vi "Encoder Motor.vi"() -> ()   [LabVIEW 2020]
uses:
  <vilib>/DAQmx/read.llb/DAQmx Read (Counter DBL 1Chan 1Samp).vi
  <vilib>/DAQmx/write.llb/DAQmx Write (Counter Frequency 1Chan 1Samp).vi
  <vilib>/DAQmx/create/channels.llb/DAQmx Create Channel (CI-Position-Angular Encoder).vi
  <vilib>/DAQmx/create/channels.llb/DAQmx Create Channel (CO-Pulse Generation-Frequency).vi
  <vilib>/DAQmx/configure/timing.llb/DAQmx Timing (Implicit).vi
  <vilib>/DAQmx/miscellaneous.llb/DAQmx Fill In Error Info.vi
  <resource>/objmgr/daqmx.rc
panel:
  out "Duty Cycle":dbl
  out "Gearbox RPM":dbl
  out "Within Range":bool
  out "Waveform Chart":dbl(graph)=3538.0740745250973
  in  "Encoder Input Counter":tag="Dev1/ctr1"
  in  "PWM Output counter":tag="Dev1/ctr0"
  out "Motor RPM":dbl
  in  "Desired RPM":dbl
  in  "stop":bool
  in  "PWM output terminal":tag="/Dev1/PFI0"
  in  "Encoder B input":tag="/Dev1/PFI9"
  in  "Encoder A input":tag="/Dev1/PFI8"
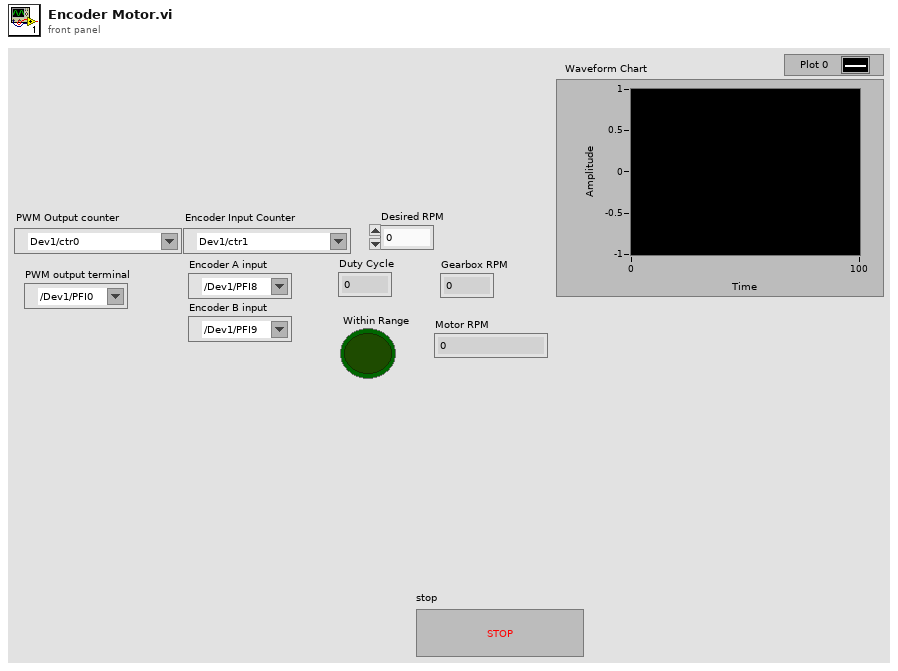
[diagram p1: front panel]
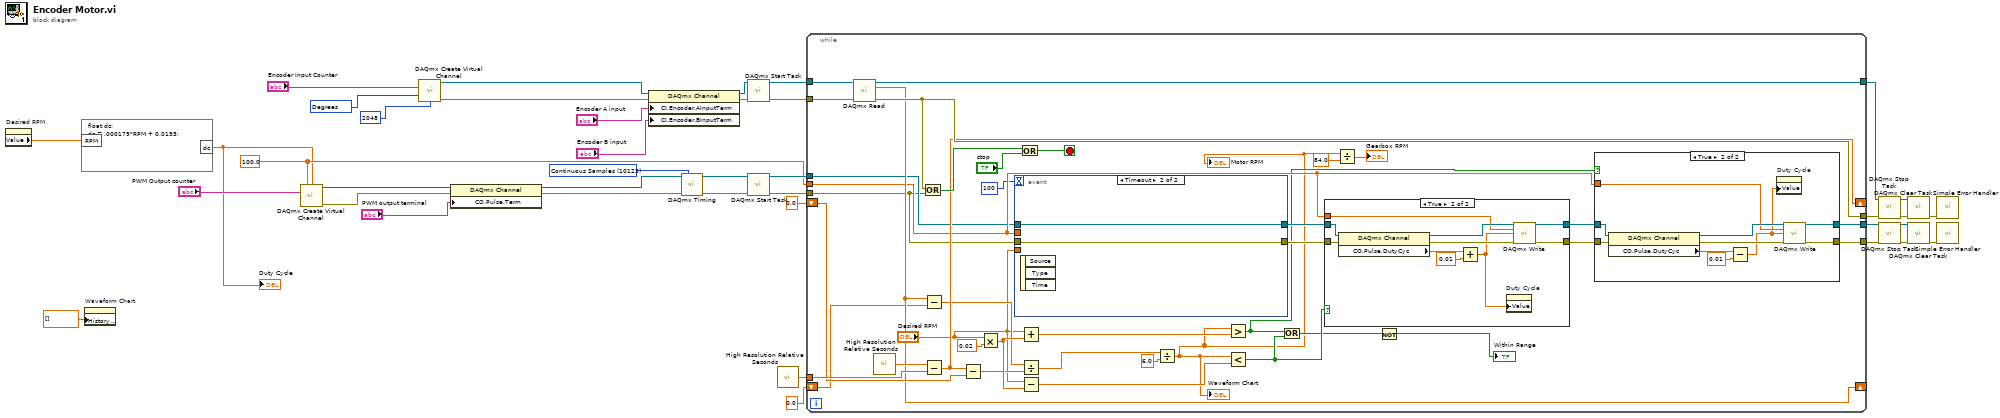
[diagram p0: block diagram]
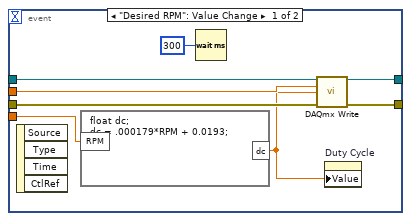
[diagram p4: hidden frame]
diagram:
  w8 = 10146 items=["Degrees"=10146, "Radians"=10273, "Ticks"=10304, "From Custom Scale"=10065] ("units")
  w14 = 10123 items=["Finite Samples"=10178, "Continuous Samples"=10123, "Hardware Timed Single Point"=12522] ("sample mode")
  w6 = 100.0 ("frequency")
  n1 = property on="Desired RPM" class="DigNum (strict)"() -> ("Value"=w3:dbl)  [unwired: 2 in, 2 out]
  n2 = formula code="float dc;\ndc = .000179*RPM + 0.0193;"("RPM"=w3) -> ("dc"=w2:dbl)
  "Duty Cycle" <- w2
  n3 = property on="Waveform Chart" class="WFChart (strict)"("History Data"=dbl[] []) -> ()  [unwired: 2 in, 2 out]
  n4 = call-poly <vilib>:"DAQmx Create Virtual Channel.vi"("frequency"=w6, "duty cycle"=w2, "counter"="PWM Output counter") -> ("task out"=w37:refnum<k21>, "error out"=w36:errorcluster)  [unwired: 11 in]
  n5 = call-poly <vilib>:"DAQmx Create Virtual Channel.vi"("counter"="Encoder Input Counter", "units"=w8, "pulses per revolution"=u32 2048) -> ("task out"=w39:refnum<k21>, "error out"=w38:errorcluster)  [unwired: 11 in]
  n6 = property class="DAQmx Channel"(reference=w37, error in=w36, "CO.Pulse.Term"="PWM output terminal") -> (reference out=w18:refnum<k21>, error out=w17:errorcluster)
  n7 = property class="DAQmx Channel"(reference=w39, error in=w38, "CI.Encoder.AInputTerm"="Encoder A input", "CI.Encoder.BInputTerm"="Encoder B input") -> (reference out=w12:refnum<k21>, error out=w11:errorcluster)
  n8 = call-poly <vilib>:"DAQmx Timing.vi"("task/channels in"=w18, "sample mode"=w14, "error in"=w17) -> ("task out"=w16:refnum<k21>, "error out"=w15:errorcluster)  [unwired: 11 in]
  n9 = call <vilib>:"DAQmx Start Task.vi"("task/channels in"=w12, "error in"=w11) -> ("task out"=w10:refnum<k21>, "error out"=w9:errorcluster)  [unwired: 12 in]
  n10 = call <vilib>:"DAQmx Start Task.vi"("task/channels in"=w16, "error in"=w15) -> ("task out"=w32:refnum<k21>, "error out"=w31:errorcluster)  [unwired: 12 in]
  n11 = call <vilib>:"High Resolution Relative Seconds.vi"() -> ("relative seconds"=w13:dbl)
  n12 = while {
    tunnel: w32 -> [w54]
    tunnel: w31 -> [w53]
    tunnel: w10 -> [w78]
    tunnel: w9 -> [w77]
    tunnel: [w65] -> w30
    tunnel: [w64] -> w29
    tunnel: [w76] -> w21
    tunnel: [w75] -> w22
    tunnel: w13 -> [w70]
    tunnel: w6 -> [w55]
    shift-right: [w62] -> _
    shift-left: 0.0 -> [w63]
    shift-right: [w61] -> _
    shift-left: 0.0 ("data") -> [w60]
    stop <- w72 stop-if-true
    n13 = call-poly <vilib>:"DAQmx Read.vi"("task/channels in"=w78, "error in"=w77) -> ("task out"=w76:refnum<k21>, "data"=w61:dbl, "error out"=w75:errorcluster)  [unwired: 11 in]
    n14 = call <vilib>:"High Resolution Relative Seconds.vi"() -> ("relative seconds"=w71:dbl)
    n15 = Or(x=w75, y=w53) -> (x .or. y?=w74:bool)
    n16 = Subtract(x=w61, y=w60) -> (x-y=w58:dbl)
    n17 = Subtract(x=w71, y=w70) -> (x-y=w62:dbl)
    n18 = Subtract(x=w62, y=w63) -> (x-y=w59:dbl)
    n19 = Multiply(x="Desired RPM", y=0.02) -> (x*y=w68:dbl)
    n20 = event shown="[1] Timeout" {
      selector: _ -> [_ _]
      dyn-events: _ -> [_ _]
      timeout: 100 -> [_ _]
      tunnel: w55 -> [w110 _]
      tunnel: w54 -> [w109 w112]
      tunnel: w53 -> [w108 w111]
      tunnel: [w107 w112] -> w52
      tunnel: [w106 w111] -> w51
      tunnel: "Desired RPM" -> [w105 _]
      event "Desired RPM": Value Change {
        n21 = event-data() -> ()  [unwired: 1 in, 4 out]
        n22 = formula code="float dc;\ndc = .000179*RPM + 0.0193;"("RPM"=w105) -> ("dc"=w103:dbl)
        n23 = Wait (ms)(milliseconds to wait=u32 300) -> ()  [unwired: 1 out]
        n24 = call-poly <vilib>:"DAQmx Write.vi"("task/channels in"=w109, "frequency"=w110, "duty cycle"=w103, "error in"=w108) -> ("task out"=w107:refnum<k21>, "error out"=w106:errorcluster)  [unwired: 9 in, 1 out]
        n25 = property on="Duty Cycle" class="DigNum (strict)"("Value"=w103) -> ()  [unwired: 2 in, 2 out]
      }
      event Timeout {
        n26 = event-data() -> ()  [unwired: 1 in, 3 out]
      }
    }
    n27 = Or(x=w74, y="stop") -> (x .or. y?=w72:bool)
    n28 = Add(x="Desired RPM", y=w68) -> (x+y=w67:dbl)
    n29 = Divide(x=w58, y=w59) -> (x/y=w57:dbl)
    n30 = Subtract(x="Desired RPM", y=w68) -> (x-y=w66:dbl)
    n31 = Divide(x=w57, y=6.0) -> (x/y=w43:dbl)
    "Motor RPM" <- w43
    "Waveform Chart" <- w43
    n32 = Greater?(x=w43, y=w67) -> (0:w45:bool)
    n33 = Less?(x=w43, y=w66) -> (x < y?=w46:bool)
    n34 = Or(x=w45, y=w46) -> (x .or. y?=w44:bool)
    n35 = case shown="True" w46 {
      tunnel: [w92 w102] -> w47
      tunnel: [w91 w101] -> w48
      tunnel: w55 -> [_ w96]
      tunnel: w52 -> [w92 w95]
      tunnel: w51 -> [w91 w94]
      frame False {
      }
      frame True {
        n36 = property class="DAQmx Channel"(reference=w95, error in=w94) -> (reference out=w100:refnum<k21>, error out=w99:errorcluster, "CO.Pulse.DutyCyc"=w97:dbl)
        n37 = Add(x=w97, y=0.01) -> (x+y=w93:dbl)
        n38 = property on="Duty Cycle" class="DigNum (strict)"("Value"=w93) -> ()  [unwired: 2 in, 2 out]
        n39 = call-poly <vilib>:"DAQmx Write.vi"("task/channels in"=w100, "frequency"=w96, "duty cycle"=w93, "error in"=w99) -> ("task out"=w102:refnum<k21>, "error out"=w101:errorcluster)  [unwired: 9 in, 1 out]
      }
    }
    n40 = Divide(x=w43, y=84.0) -> (x/y=→"Gearbox RPM":dbl)
    n41 = Not(x=w44) -> (.not. x?=→"Within Range":bool)
    n42 = case shown="True" w45 {
      tunnel: w48 -> [w79 w88]
      tunnel: w47 -> [w80 w87]
      tunnel: [w80 w86] -> w65
      tunnel: [w79 w85] -> w64
      tunnel: w55 -> [_ w84]
      frame False {
      }
      frame True {
        n43 = property class="DAQmx Channel"(reference=w87, error in=w88) -> (reference out=w90:refnum<k21>, error out=w89:errorcluster, "CO.Pulse.DutyCyc"=w82:dbl)
        n44 = Subtract(x=w82, y=0.01) -> (x-y=w81:dbl)
        n45 = property on="Duty Cycle" class="DigNum (strict)"("Value"=w81) -> ()  [unwired: 2 in, 2 out]
        n46 = call-poly <vilib>:"DAQmx Write.vi"("task/channels in"=w90, "frequency"=w84, "duty cycle"=w81, "error in"=w89) -> ("task out"=w86:refnum<k21>, "error out"=w85:errorcluster)  [unwired: 9 in, 1 out]
      }
    }
  }
  n47 = call <vilib>:"DAQmx Stop Task.vi"("task/channels in"=w21, "error in"=w22) -> ("task out"=w25:refnum<k21>, "error out"=w24:errorcluster)  [unwired: 12 in]
  n48 = call <vilib>:"DAQmx Stop Task.vi"("task/channels in"=w30, "error in"=w29) -> ("task out"=w28:refnum<k21>, "error out"=w27:errorcluster)  [unwired: 12 in]
  n49 = call <vilib>:"DAQmx Clear Task.vi"("task in"=w25, "error in"=w24) -> ("error out"=w23:errorcluster)  [unwired: 13 in]
  n50 = call <vilib>:"DAQmx Clear Task.vi"("task in"=w28, "error in"=w27) -> ("error out"=w26:errorcluster)  [unwired: 13 in]
  n51 = call <vilib>:"Simple Error Handler.vi"("error in (no error)"=w23) -> ()  [unwired: 4 in, 5 out]
  n52 = call <vilib>:"Simple Error Handler.vi"("error in (no error)"=w26) -> ()  [unwired: 4 in, 5 out]
